vi "Data Socket mio reader.vi"(1 "stop":bool, 2 "String":string) -> (0 "Indicatore":dbl)   [LabVIEW 2012]
panel:
  # "Default:\n\nlocalhost/samplenum"
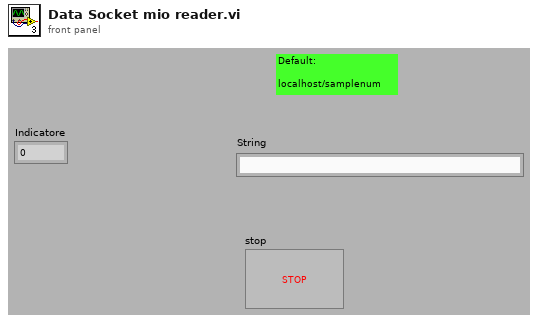
[diagram p1: front panel]
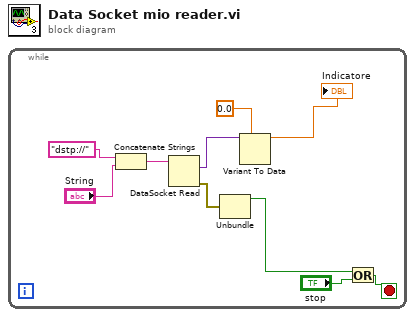
[diagram p0: block diagram]
diagram:
  n1 = while {
    stop <- w7 stop-if-true
    n2 = Concatenate Strings("dstp://" ("connection in"), "String") -> (w1:string)
    n3 = DataSocket Read(11:w1) -> (0:w10:errorcluster, 2:w6:variant)  [unwired: 4 in, 5 out]
    n4 = Unbundle(w10) -> ("status"=w9:bool)  [unwired: 2 out]
    n5 = Variant To Data(type=0.0, Variant=w6) -> (data=→"Indicatore":dbl)  [unwired: 1 in, 1 out]
    n6 = Or(x=w9, y="stop") -> (x .or. y?=w7:bool)
  }
